vi "LVPortConvertObjectMapTypeName.vi"(10 "TypeName":string, 11 "ObjectMapType in":T1) -> (2 "Typename":string, 3 "ObjectMapType out":T1)   [LabVIEW 2017]
uses:
  LVPortObjectMapDataTypeEnum.ctl
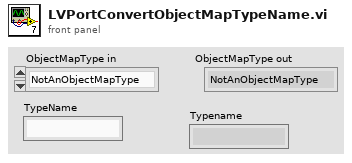
[diagram p1: front panel]
types:
  T1 = typedef "LVPortObjectMapDataTypeEnum.ctl" = enum16{"NotAnObjectMapType", "Real", "Complex", "String", "Boolean"}
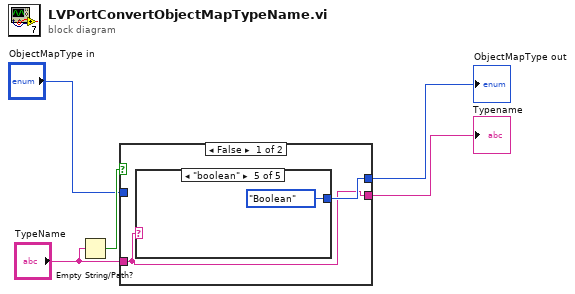
[diagram p0: block diagram]
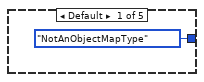
[diagram p2: hidden frame]
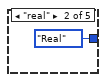
[diagram p3: hidden frame]
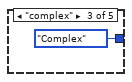
[diagram p4: hidden frame]
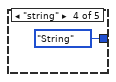
[diagram p5: hidden frame]
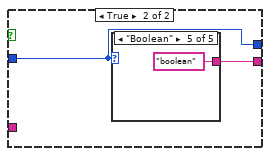
[diagram p6: hidden frame]
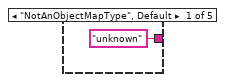
[diagram p7: hidden frame]
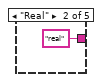
[diagram p8: hidden frame]
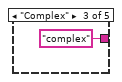
[diagram p9: hidden frame]
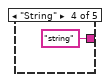
[diagram p10: hidden frame]
diagram:
  n1 = Empty String/Path?(string/path="TypeName") -> (empty?=w3:bool)
  n2 = case shown="False" w3 {
    tunnel: "ObjectMapType in" -> [_ w13]
    tunnel: [w6 w14] -> w2
    tunnel: "TypeName" -> [w6 _]
    tunnel: [w7 w13] -> w5
    frame False {
      n3 = case shown="\"boolean\"" w6 {
        tunnel: [LVPortObjectMapDataTypeEnum."NotAnObjectMapType" ("MatlabType") LVPortObjectMapDataTypeEnum."Real" ("MatlabType") LVPortObjectMapDataTypeEnum."Complex" ("MatlabType") LVPortObjectMapDataTypeEnum."String" ("MatlabType") LVPortObjectMapDataTypeEnum."Boolean" ("MatlabType")] -> w7
        frame Default {
        }
        frame "real" {
        }
        frame "complex" {
        }
        frame "string" {
        }
        frame "boolean" {
        }
      }
    }
    frame True {
      n4 = case shown="\"Boolean\"" w13 {
        tunnel: ["unknown" ("Typename") "real" ("Typename") "complex" ("Typename") "string" ("Typename") "boolean" ("Typename")] -> w14
        frame "NotAnObjectMapType", Default {
        }
        frame "Real" {
        }
        frame "Complex" {
        }
        frame "String" {
        }
        frame "Boolean" {
        }
      }
    }
  }
  "ObjectMapType out" <- w5
  "Typename" <- w2
